vi "Initialize.vi"(8 "error in (no error)":errorcluster, 11 "S4ACS_GUI in":refnum<class "S4ACS_GUI.lvclass">) -> (0 "error out":errorcluster, 3 "S4ACS_GUI out":refnum<class "S4ACS_GUI.lvclass">)   [LabVIEW 2018, in "S4ACS_GUI.lvclass"]
uses:
  S4ACS_GUI.lvclass
  S4ACS_GUI.lvclass/S4ACS_GUI.ctl
  Acquisition/Acquisition.lvclass
  Instrument/Instrument.lvclass
  SyncBox/Sync Box.lvclass
  SetupFile/Setup File.lvclass
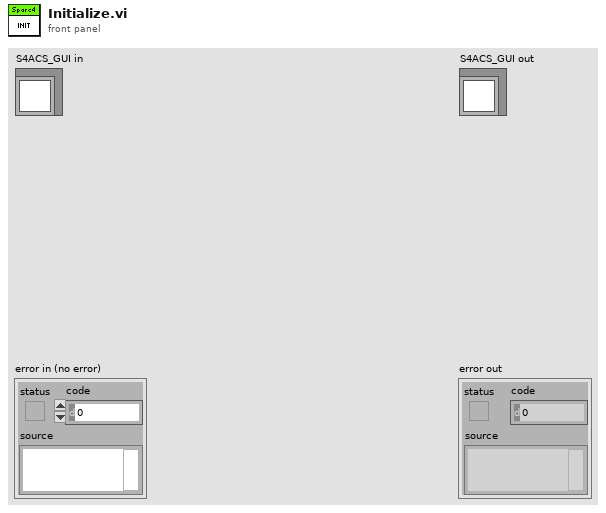
[diagram p1: front panel]
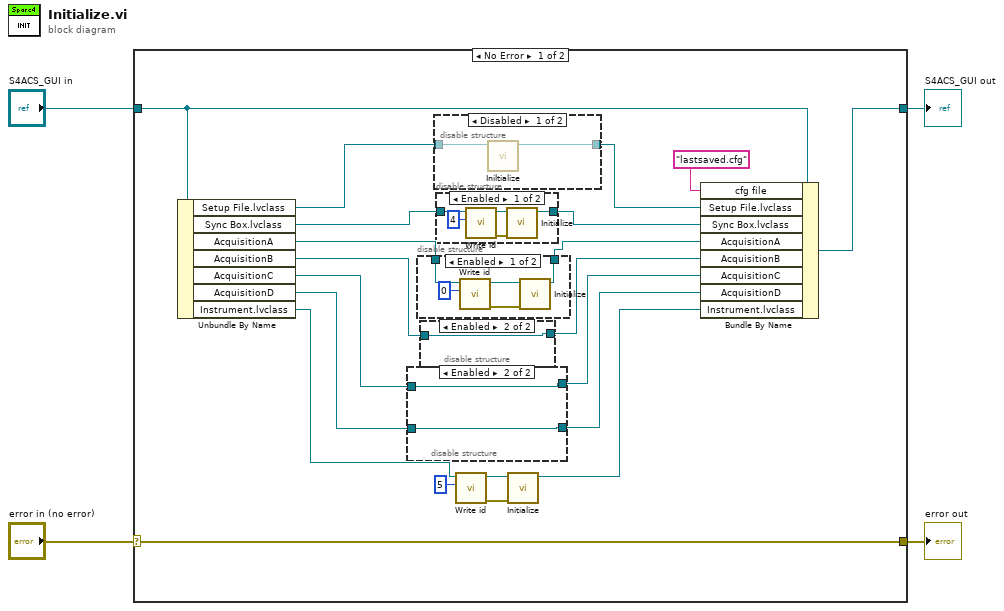
[diagram p0: block diagram]
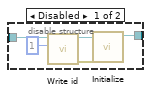
[diagram p2: hidden frame]
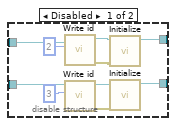
[diagram p3: hidden frame]
diagram:
  n1 = case shown="No Error" "error in (no error)" {
    selector: "error in (no error)" -> [w19 w60]
    tunnel: [w19 w60] -> w3
    tunnel: [w6 w59] -> w1
    tunnel: "S4ACS_GUI in" -> [w7 w59]
    frame No Error {
      n2 = Unbundle By Name(w7) -> ("Setup File.lvclass"=w25:refnum<class "Setup File.lvclass">, "Sync Box.lvclass"=w13:refnum<class "Sync Box.lvclass">, "AcquisitionA"=w21:refnum<class "Acquisition.lvclass">, "AcquisitionB"=w20:refnum<class "Acquisition.lvclass">, "AcquisitionC"=w18:refnum<class "Acquisition.lvclass">, "AcquisitionD"=w17:refnum<class "Acquisition.lvclass">, "Instrument.lvclass"=w9:refnum<class "Instrument.lvclass">)
      n3 = disable-structure shown="Enabled" {
        disable-tunnel: w18 -> [w41 w43]
        disable-tunnel: w17 -> [w40 w42]
        disable-tunnel: [w39 w43] -> w16
        disable-tunnel: [w38 w42] -> w15
        frame Disabled {
          n4 = call-dynamic "Write id.vi"("id"=u32 2, "Server in"=w41) -> ("error out"=w35:errorcluster, "Server out"=w34:refnum<class "Acquisition.lvclass">)  [unwired: 8 in]
          n5 = call-dynamic "Write id.vi"("id"=u32 3, "Server in"=w40) -> ("error out"=w32:errorcluster, "Server out"=w36:refnum<class "Acquisition.lvclass">)  [unwired: 8 in]
          n6 = call-dynamic "Initialize.vi"("error in (no error)"=w35, "Acquisition in"=w34) -> ("Acquisition out"=w39:refnum<class "Acquisition.lvclass">)  [unwired: 8 in, 1 out]
          n7 = call-dynamic "Initialize.vi"("error in (no error)"=w32, "Acquisition in"=w36) -> ("Acquisition out"=w38:refnum<class "Acquisition.lvclass">)  [unwired: 8 in, 1 out]
        }
        frame Enabled {
        }
      }
      n8 = disable-structure shown="Enabled" {
        disable-tunnel: [w48 w49] -> w23
        disable-tunnel: w21 -> [w47 w49]
        frame Enabled {
          n9 = call-dynamic "Write id.vi"("id"=u32 0, "Server in"=w47) -> ("error out"=w44:errorcluster, "Server out"=w45:refnum<class "Acquisition.lvclass">)  [unwired: 8 in]
          n10 = call-dynamic "Initialize.vi"("error in (no error)"=w44, "Acquisition in"=w45) -> ("Acquisition out"=w48:refnum<class "Acquisition.lvclass">)  [unwired: 8 in, 1 out]
        }
        frame Disabled {
        }
      }
      n11 = disable-structure shown="Enabled" {
        disable-tunnel: [w30 w31] -> w22
        disable-tunnel: w20 -> [w29 w31]
        frame Disabled {
          n12 = call-dynamic "Write id.vi"("id"=u32 1, "Server in"=w29) -> ("error out"=w26:errorcluster, "Server out"=w28:refnum<class "Acquisition.lvclass">)  [unwired: 8 in]
          n13 = call-dynamic "Initialize.vi"("error in (no error)"=w26, "Acquisition in"=w28) -> ("Acquisition out"=w30:refnum<class "Acquisition.lvclass">)  [unwired: 8 in, 1 out]
        }
        frame Enabled {
        }
      }
      n14 = disable-structure shown="Disabled" {
        disable-tunnel: w25 -> [w56 w58]
        disable-tunnel: [w57 w58] -> w24
        frame Disabled {
          n15 = call-dynamic "Iniltialize.vi"("Setup File in"=w56) -> ("Setup File out"=w57:refnum<class "Setup File.lvclass">)  [unwired: 9 in, 1 out]
        }
        frame Enabled {
        }
      }
      n16 = disable-structure shown="Enabled" {
        disable-tunnel: [w54 w55] -> w14
        disable-tunnel: w13 -> [w53 w55]
        frame Enabled {
          n17 = call-dynamic "Write id.vi"("id"=u32 4, "Server in"=w53) -> ("error out"=w50:errorcluster, "Server out"=w51:refnum<class "Sync Box.lvclass">)  [unwired: 8 in]
          n18 = call-dynamic "Initialize.vi"("error in (no error)"=w50, "Sync Box in"=w51) -> ("Sync Box out"=w54:refnum<class "Sync Box.lvclass">)  [unwired: 8 in, 1 out]
        }
        frame Disabled {
        }
      }
      n19 = call-dynamic "Write id.vi"("id"=u32 5, "Server in"=w9) -> ("error out"=w10:errorcluster, "Server out"=w11:refnum<class "Instrument.lvclass">)  [unwired: 8 in]
      n20 = call-dynamic "Initialize.vi"("error in (no error)"=w10, "Instrument in"=w11) -> ("Instrument out"=w8:refnum<class "Instrument.lvclass">)  [unwired: 8 in, 1 out]
      n21 = Bundle By Name(cluster=w7, "cfg file"="lastsaved.cfg", "Setup File.lvclass"=w24, "Sync Box.lvclass"=w14, "AcquisitionA"=w23, "AcquisitionB"=w22, "AcquisitionC"=w16, "AcquisitionD"=w15, "Instrument.lvclass"=w8) -> (w6:refnum<class "S4ACS_GUI.lvclass">)
    }
    frame Error {
    }
  }
  "error out" <- w3
  "S4ACS_GUI out" <- w1
